vi "macro_PhotonVision_PoseEstimatorExecClosestToLastPose.vi"() -> ()   [LabVIEW 2019]
uses:
  <vilib>/Rock Robotics/WPI/ThirdParty/JAS_Junk/TrajLib/TypeDef/POSE3D.ctl
  <vilib>/Rock Robotics/WPI/ThirdParty/JAS_Junk/TrajLib/TypeDef/TRANSLATION3D.ctl
  <vilib>/Rock Robotics/WPI/ThirdParty/JAS_Junk/TrajLib/TypeDef/ROTATION3D.ctl
  <vilib>/Rock Robotics/WPI/ThirdParty/JAS_Junk/TrajLib/TypeDef/QUATERNION.ctl
  PhotonVisionLib/Enum/PhotonPoseStrategy_ENUM.ctl
  <vilib>/Rock Robotics/WPI/ThirdParty/JAS_Junk/TrajLib/VI/AprilTagFieldLayout_New.vi
  <vilib>/Rock Robotics/WPI/ThirdParty/JAS_Junk/TrajLib/VI/Quaternion_New.vi
  <vilib>/Rock Robotics/WPI/ThirdParty/JAS_Junk/TrajLib/VI/Pose3d_New_Trans3dRot3d.vi
  <vilib>/Rock Robotics/WPI/ThirdParty/JAS_Junk/TrajLib/VI/Rotation3d_Create_Quaternion.vi
  <vilib>/Rock Robotics/WPI/ThirdParty/JAS_Junk/TrajLib/VI/AprilTag_New.vi
  <vilib>/Rock Robotics/WPI/ThirdParty/JAS_Junk/TrajLib/Conv_Deg_Radians.vi
  PhotonVisionLib/SubVI/PhotonPipelineResult_Unpack.vi
  PhotonVisionLib/SubVI/PhotonPipelineResult_GetTargetCount.vi
  PhotonVisionLib/SubVI/PhotonPipelineResult_GetMetadata.vi
  PhotonVisionLib/SubVI/PhotonPipelineMetadata_GetAll.vi
  <vilib>/Rock Robotics/WPI/ThirdParty/JAS_Junk/TrajLib/VI/Transform3d_Equals.vi
  PhotonVisionLib/SubVI/PhotonPoseEstimator_SetCamera.vi
  PhotonVisionLib/SubVI/PhotonPoseEstimator_SetHighestAmbiguity.vi
  PhotonVisionLib/SubVI/PhotonPoseEstimator_SetRobotToCameraTransform.vi
  PhotonVisionLib/SubVI/PhotonPoseEstimator_New.vi
  PhotonVisionLib/SubVI/PhotonPoseEstimator_SetLastPose.vi
  PhotonVisionLib/SubVI/PhotonPoseEstimator_Update_ClosestToLastPose.vi
  PhotonVisionLib/SubVI/PhotonEstimatedRobotPose_GetAll.vi
  <vilib>/Rock Robotics/WPI/ThirdParty/JAS_Junk/TrajLib/VI/Pose3d_ToPose2d.vi
  <vilib>/Rock Robotics/WPI/ThirdParty/JAS_Junk/TrajLib/VI/AprilTag_GetAll.vi
  <vilib>/Rock Robotics/WPI/ThirdParty/JAS_Junk/TrajLib/VI/Quaternion_Normalize.vi
  PhotonVisionLib/SubVI/Packet_decode_ByteI8.vi
  PhotonVisionLib/SubVI/PhotonTrackedTarget_Unpack.vi
  PhotonVisionLib/SubVI/PhotonMultiTargetPNPResult_unpack.vi
  PhotonVisionLib/SubVI/PhotonPipelineMetadata_Unpack.vi
  PhotonVisionLib/SubVI/PhotonPipelineResult_New.vi
  <vilib>/Rock Robotics/WPI/ThirdParty/JAS_Junk/TrajLib/VI/Transform3d_GetTranslation3d.vi
  <vilib>/Rock Robotics/WPI/ThirdParty/JAS_Junk/TrajLib/VI/Transform3d_GetRotation3d.vi
  <vilib>/Rock Robotics/WPI/ThirdParty/JAS_Junk/TrajLib/VI/Rotation3d_Equals.vi
  <vilib>/Rock Robotics/WPI/ThirdParty/JAS_Junk/TrajLib/VI/Translation3d_Equals.vi
  PhotonVisionLib/SubVI/PhotonTargetModel_New_AprilTag36H11.vi
  <vilib>/Rock Robotics/WPI/ThirdParty/JAS_Junk/TrajLib/VI/TimeInterpRotation2d_New.vi
  PhotonVisionLib/SubVI/PhotonPoseEstimator_GetEmptyPose.vi
  PhotonVisionLib/SubVI/PhotonPoseEstimator_EstimateClosestToLastPose.vi
  PhotonVisionLib/SubVI/PhotonPoseEstimator_GetLastPose.vi
  PhotonVisionLib/SubVI/PhotonPipelineResult_GetTimeStampSecs.vi
  <vilib>/Rock Robotics/WPI/ThirdParty/JAS_Junk/TrajLib/VI/Pose3d_getTranslation3d.vi
  <vilib>/Rock Robotics/WPI/ThirdParty/JAS_Junk/TrajLib/VI/Pose3d_getRotation3d.vi
  <vilib>/Rock Robotics/WPI/ThirdParty/JAS_Junk/TrajLib/VI/Translation3d_ToTranslation2d.vi
  <vilib>/Rock Robotics/WPI/ThirdParty/JAS_Junk/TrajLib/VI/Rotation3d_ToRotation2d.vi
  <vilib>/Rock Robotics/WPI/ThirdParty/JAS_Junk/TrajLib/Pose2d_New_TRRO.vi
  <vilib>/Rock Robotics/WPI/ThirdParty/JAS_Junk/TrajLib/VI/Quaternion_New_Default.vi
  PhotonVisionLib/SubVI/Packet_decode_Flt64.vi
  PhotonVisionLib/SubVI/TargetCorner_New.vi
  PhotonVisionLib/SubVI/Packet_decode_Int32.vi
  PhotonVisionLib/SubVI/Packet_decode_Transform3d.vi
  PhotonVisionLib/SubVI/Packet_decode_Flt32.vi
  PhotonVisionLib/SubVI/Packet_decode_TargetCornerArray.vi
  PhotonVisionLib/SubVI/Packet_decode_Boolean.vi
  PhotonVisionLib/SubVI/PhotonPNPResult_unpack.vi
  PhotonVisionLib/SubVI/PhotonMultiTargetPNPResult_New.vi
  PhotonVisionLib/SubVI/Packet_decode_Int16.vi
  PhotonVisionLib/SubVI/Packet_decode_Int64.vi
  <vilib>/Rock Robotics/WPI/ThirdParty/JAS_Junk/TrajLib/VI/Rotation3d_GetQuaterion.vi
  <vilib>/Rock Robotics/WPI/ThirdParty/JAS_Junk/TrajLib/VI/Quaternion_Equals.vi
  PhotonVisionLib/SubVI/PhotonTargetModel_New_RectPlanar.vi
  <vilib>/Rock Robotics/WPI/ThirdParty/JAS_Junk/TrajLib/Conv_Inches_Meters.vi
  <vilib>/Rock Robotics/WPI/ThirdParty/JAS_Junk/TrajLib/VI/Rotation3d_Create_AxisAngle.vi
  <vilib>/Rock Robotics/WPI/ThirdParty/JAS_Junk/TrajLib/VI/Pose3d_New.vi
  PhotonVisionLib/SubVI/PhotonPipelineResult_HasTargets.vi
  PhotonVisionLib/SubVI/PhotonEstimatedRobotPose_New.vi
  PhotonVisionLib/SubVI/PhotonPipelineResult_GetTargets.vi
  <vilib>/Rock Robotics/WPI/ThirdParty/JAS_Junk/TrajLib/VI/AprilTagFieldLayout_GetTagPose.vi
  PhotonVisionLib/SubVI/PhotonTrackedTarget_GetFiducialId.vi
  PhotonVisionLib/SubVI/PhotonTrackedTarget_GetAltCameraToTarget.vi
  PhotonVisionLib/SubVI/PhotonTrackedTarget_GetBestCameraToTarget.vi
  PhotonVisionLib/SubVI/PhotonPoseEstimator_Strategy_closestToReferencePose_calc.vi
  PhotonVisionLib/SubVI/PhotonTrackedTarget_GetPoseAmbiguity.vi
  PhotonVisionLib/SubVI/PhotonPoseEstimator_GetFieldTags.vi
  PhotonVisionLib/SubVI/PhotonPoseEstimator_GetRobotToCameraTransform.vi
  PhotonVisionLib/SubVI/PhotonPoseEstimator_GetHighestAmbiguity.vi
  <vilib>/Rock Robotics/WPI/ThirdParty/JAS_Junk/TrajLib/Translation2d_Create.vi
  <vilib>/Rock Robotics/WPI/ThirdParty/JAS_Junk/TrajLib/Rotation2d_CreateAngle.vi
  <vilib>/Rock Robotics/WPI/ThirdParty/JAS_Junk/TrajLib/VI/Rotation3d_GetXYZ.vi
  PhotonVisionLib/SubVI/PhotonPNPResult_New.vi
  <vilib>/Rock Robotics/WPI/ThirdParty/JAS_Junk/TrajLib/VI/Quaternion_Get_Vect.vi
  <vilib>/Rock Robotics/WPI/ThirdParty/JAS_Junk/TrajLib/VI/Quaternion_Get_W.vi
  PhotonVisionLib/SubVI/PhotonTargetModel_New.vi
  <vilib>/Rock Robotics/WPI/ThirdParty/JAS_Junk/TrajLib/VI/Rotation3d_Create_Default.vi
  <vilib>/Rock Robotics/WPI/ThirdParty/JAS_Junk/TrajLib/VI/Vector_Norm.vi
  <vilib>/Rock Robotics/WPI/ThirdParty/JAS_Junk/TrajLib/VecBuilder_ArrayBy1Fill.vi
  <vilib>/Rock Robotics/WPI/ThirdParty/JAS_Junk/TrajLib/VI/Pose3d_RelativeTo.vi
  <vilib>/Rock Robotics/WPI/ThirdParty/JAS_Junk/TrajLib/Transform2d_Create_TransRot.vi
  <vilib>/Rock Robotics/WPI/ThirdParty/JAS_Junk/TrajLib/VI/Pose3d_TransformBy.vi
  <vilib>/Rock Robotics/WPI/ThirdParty/JAS_Junk/TrajLib/VI/Transform3d_Inverse.vi
  PhotonVisionLib/SubVI/PhotonPoseEstimator_CalcDifference.vi
  <vilib>/Rock Robotics/WPI/ThirdParty/JAS_Junk/TrajLib/VI/Quaternion_Get_All.vi
  <vilib>/Rock Robotics/WPI/ThirdParty/JAS_Junk/TrajLib/MatBuilder_Create.vi
  <vilib>/Rock Robotics/WPI/ThirdParty/JAS_Junk/TrajLib/VI/Transform3d_Create_Pose3dPose3d.vi
  <vilib>/Rock Robotics/WPI/ThirdParty/JAS_Junk/TrajLib/VI/Translation3d_Plus.vi
  <vilib>/Rock Robotics/WPI/ThirdParty/JAS_Junk/TrajLib/VI/Translation3d_RotateBy.vi
  <vilib>/Rock Robotics/WPI/ThirdParty/JAS_Junk/TrajLib/VI/Rotation3d_Plus.vi
  <vilib>/Rock Robotics/WPI/ThirdParty/JAS_Junk/TrajLib/VI/Rotation3d_UnaryMinus.vi
  <vilib>/Rock Robotics/WPI/ThirdParty/JAS_Junk/TrajLib/VI/Translation3d_UnaryMinus.vi
  <vilib>/Rock Robotics/WPI/ThirdParty/JAS_Junk/TrajLib/VI/Translation3d_GetDistance.vi
  <vilib>/Rock Robotics/WPI/ThirdParty/JAS_Junk/TrajLib/VI/Translation3d_Minus.vi
  <vilib>/Rock Robotics/WPI/ThirdParty/JAS_Junk/TrajLib/VI/Rotation3d_Minus.vi
  <vilib>/Rock Robotics/WPI/ThirdParty/JAS_Junk/TrajLib/VI/Quaternion_Times.vi
  <vilib>/Rock Robotics/WPI/ThirdParty/JAS_Junk/TrajLib/VI/Quaternion_Inverse.vi
  <vilib>/Rock Robotics/WPI/ThirdParty/JAS_Junk/TrajLib/VI/Rotation3d_RotateBy.vi
  <vilib>/Rock Robotics/Network Tables/NT Read Value.vi
  <vilib>/Rock Robotics/Network Tables/NT Read Raw.vi
  PhotonVisionLib/PhotonVisionLib.lvlib
  <vilib>/Rock Robotics/WPI/ThirdParty/JAS_Junk/TrajLib/Trajectory_Library.lvlib
  <vilib>/Rock Robotics/WPI/ThirdParty/JAS_Junk/TrajLib/VI/AprilTagFieldLayout_New2026Welded.vi
panel:
  out "TimeStamp_Seconds":dbl
  out "EstimatedPose3d":T1={"Translation3d"={"X"=0.0, "Y"=0.0, "Z"=0.0}, "Rotation3d"={"Q_quaternion"={"R"=1.0, "V"=[0.0, 0.0, 0.0]}}} {"Translation3d"."Z" format="%14.3f"; "Translation3d"."Y" format="%14.3f"; "Translation3d"."X" format="%14.3f"}
  out "New Pose Found":bool
  out "IsConnected":bool
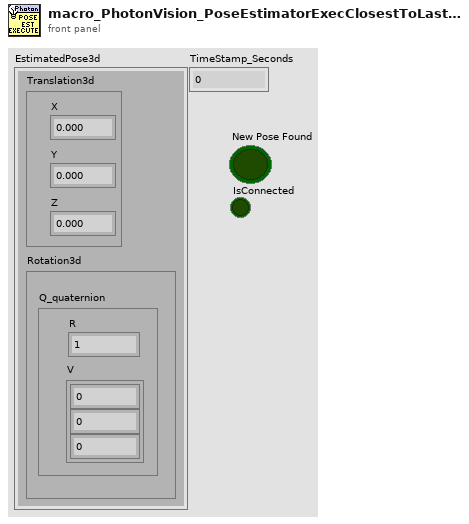
[diagram p1: front panel]
types:
  T1 = typedef "Trajectory_Library.lvlib/POSE3D.ctl" = cluster{"Translation3d":T2, "Rotation3d":T3}
  T2 = typedef "Trajectory_Library.lvlib/TRANSLATION3D.ctl" = cluster{"X":dbl, "Y":dbl, "Z":dbl}
  T3 = typedef "Trajectory_Library.lvlib/ROTATION3D.ctl" = cluster{"Q_quaternion":T4}
  T4 = typedef "Trajectory_Library.lvlib/QUATERNION.ctl" = cluster{"R":dbl, "V":dbl[]}
  T5 = typedef "PhotonVisionLib.lvlib/PhotonPoseStrategy_ENUM.ctl" = enum16{"LOWEST_AMBIGUITY", "CLOSEST_TO_CAMERA_HEIGHT", "CLOSEST_TO_REFERENCE_POSE", "CLOSEST_TO_LAST_POSE", "AVERAGE_BEST_TARGETS", "MULTI_TAG_PNP_ON_COPROCESSOR", "MULTI_TAG_PNP_ON_RIO", "PNP_DISTANCE_TRIG_SOLVE", "CONSTRAINED_SOLVEPNP"}
  T6 = typedef "Trajectory_Library.lvlib/AprilTagFieldLayout.ctl" = cluster{"AprilTagMap":map{i32, T7}, "FieldLength":dbl, "FieldWidth":dbl, "OriginPosition ":T8, "OriginPose3d":T1}
  T7 = typedef "Trajectory_Library.lvlib/AprilTag.ctl" = cluster{"ID":i32, "POSE3D":T1}
  T8 = typedef "Trajectory_Library.lvlib/AprilTagFieldLayoutOrignPosition_ENUM.ctl" = enum16{"kBlueAllianceWallRightSide,", "kRedAllianceWallRightSide,"}
  T9 = typedef "Trajectory_Library.lvlib/TRANSFORM3D.ctl" = cluster{"TRANSLATION3D":T2, "ROTATION3D":T3, "XF":bool}
  T10 = typedef "PhotonVisionLib.lvlib/PhotonPipelineResultType.ctl" = cluster{"Targets":T11[], "PhotonMultiTargetPNPResult":T13, "PhotonPipelineMetadata":T15}
  T11 = typedef "PhotonVisionLib.lvlib/PhotonTrackedTargetType.ctl" = cluster{"Yaw":dbl, "Pitch":dbl, "Area":dbl, "Skew":dbl, "MinAreaRectCorners":T12[], "BestCameraToTarget":T9, "FiducialId":i32, "AltCameraToTarget":T9, "PoseAmbiguity":dbl, "DetectedCorners":T12[], "ObjDetectId":i32, "ObjDetectConf":sgl}
  T12 = typedef "PhotonVisionLib.lvlib/TargetCornerType.ctl" = cluster{"X":dbl, "Y":dbl}
  T13 = typedef "PhotonVisionLib.lvlib/PhotonMultiTargetPNPResultType.ctl" = cluster{"PhotonPNPResult":T14, "FiducialIDsUsed":i16[]}
  T14 = typedef "PhotonVisionLib.lvlib/PhotonPNPResultType.ctl" = cluster{"IsPresent":bool, "bestReprojErr":dbl, "altReprojErr":dbl, "ambiguity":dbl, "Best":T9, "Alt":T9}
  T15 = typedef "PhotonVisionLib.lvlib/PhotonPipelineMetadataType.ctl" = cluster{"CaptureTimestampMicros":i64, "PublishTimestampMicros":i64, "SequenceID":i64, "TimeSinceLastPong":i64}
  T16 = typedef "PhotonVisionLib.lvlib/PhotonPoseEstimator_Configuration.ctl" = cluster{"Primary Strategy":T5, "Camera":string, "Initial Pose":T1, "HighestAmbiguity":dbl, "RobotToCamera":T9, "FallBack Strategy":T5, "BaseNTName":string}
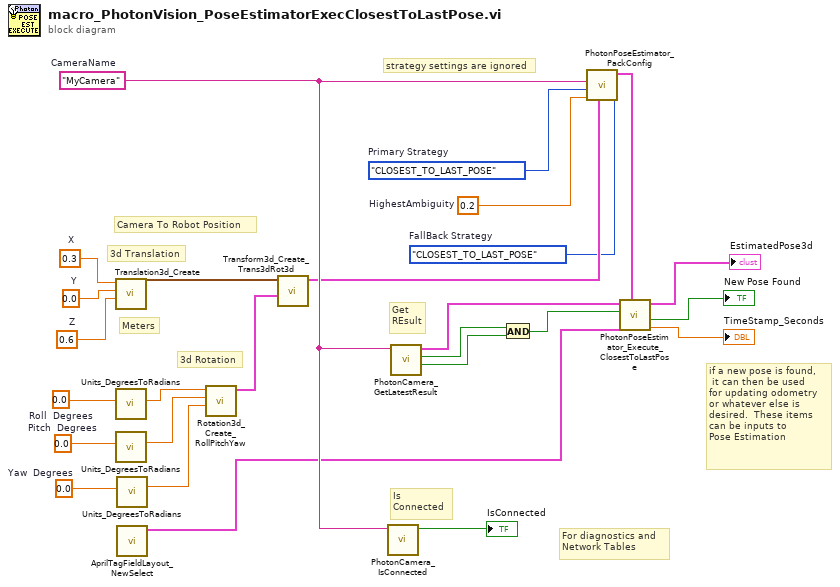
[diagram p0: block diagram]
diagram:
  w6 = PhotonPoseStrategy_ENUM."CLOSEST_TO_LAST_POSE"  # FallBack Strategy
  w14 = 0.0  # Roll  Degrees
  w15 = 0.0  # Pitch  Degrees
  w16 = 0.0  # Yaw  Degrees
  w22 = 0.6  # Z
  w21 = 0.3  # X
  w20 = 0.0  # Y
  w23 = 0.2  # HighestAmbiguity
  w24 = PhotonPoseStrategy_ENUM."CLOSEST_TO_LAST_POSE"  # Primary Strategy
  w25 = "MyCamera"  # CameraName
  # "strategy settings are ignored"
  # "For diagnostics and \nNetwork Tables"
  # "if a new pose is found, \n it can then be used\nfor updating odometry\nor whatever else is \ndesired.  These items\ncan be inputs to\nPose Estimation"
  # "Meters"
  # "Camera To Robot Position"
  # "3d Rotation"
  # "3d Translation"
  # "Is\nConnected"
  # "Get\nREsult"
  n1 = call <vilib>:"Translation3d_Create.vi"("Z"=w22, "Y"=w20, "X"=w21) -> ("TRANSLATION3D"=w13:T2)  [unwired: 8 in]
  n2 = call <vilib>:"Units_DegreesToRadians.vi"("Degrees"=w14) -> ("Radians"=w17:dbl)  [unwired: 10 in]
  n3 = call <vilib>:"Units_DegreesToRadians.vi"("Degrees"=w15) -> ("Radians"=w18:dbl)  [unwired: 10 in]
  n4 = call <vilib>:"Units_DegreesToRadians.vi"("Degrees"=w16) -> ("Radians"=w19:dbl)  [unwired: 10 in]
  n5 = call-poly <vilib>:"AprilTagFieldLayout_NewSelect.vi"() -> ("AprilTagFieldLayout"=w1:T6)  [unwired: 11 in]
  n6 = call <vilib>:"Rotation3d_Create_RollPitchYaw.vi"("Yaw"=w19, "Pitch"=w18, "Roll"=w17) -> ("Rotation3d"=w12:T3)  [unwired: 8 in]
  n7 = call <vilib>:"Transform3d_Create_Trans3dRot3d.vi"("Rotation3d"=w12, "Translation3d"=w13) -> ("Transform3d"=w11:T9)  [unwired: 9 in]
  n8 = call "PhotonCamera_IsConnected.vi"("CameraName"=w25) -> ("IsConnected"=→"IsConnected":bool)  [unwired: 9 in, 1 out]
  n9 = call "PhotonCamera_GetLatestResult.vi"("CameraName"=w25) -> ("New Data"=w7:bool, "HasTargets"=w8:bool, "PipelineResult"=w10:T10)  [unwired: 6 in, 2 out]
  n10 = And(x=w8, y=w7) -> (x .and. y?=w9:bool)
  n11 = call "PhotonPoseEstimator_PackConfig.vi"("FallBack Strategy"=w6, "RobotToCamera"=w11, "HighestAmbiguity"=w23, "PirmaryStrategy"=w24, "Camera"=w25) -> ("PoseEstimator_Configuration"=w26:T16)  [unwired: 6 in]
  n12 = call "PhotonPoseEstimator_Execute_ClosestToLastPose.vi"("Configuration"=w26, "AprilTagFieldLayout"=w1, "PIpeline Has \nNew Results"=w9, "PipelineResult"=w10) -> ("TimeStamp_Seconds"=→"TimeStamp_Seconds":dbl, "New Pose Found"=→"New Pose Found":bool, "EstimatedPose3d"=→"EstimatedPose3d":T1)  [unwired: 2 in, 3 out]
